vi "Back Right Wheel.vi"(9 "output cluster 2":T2, 10 "Pot Val in":dbl, 11 "Wheel Angle Offset":dbl) -> (0 "Wheel Angle":dbl, 1 "Drive Speed":dbl, 3 "Wheel Speed":dbl)   [LabVIEW 2019]
uses:
  <vilib>/addons/control/pid/pid.llb/PID (DBL).vi
  <vilib>/addons/control/pid/NI_PID_pid.lvlib
panel:
  in  "PID gains":T1={"proportional gain (Kc)"=0.01, "integral time (Ti, min)"=0.0, "derivative time (Td, min)"=0.0} {"derivative time (Td, min)" format="%.3f"; "integral time (Ti, min)" format="%.3f"; "proportional gain (Kc)" format="%.3f"}
  out "Requested Angle":dbl
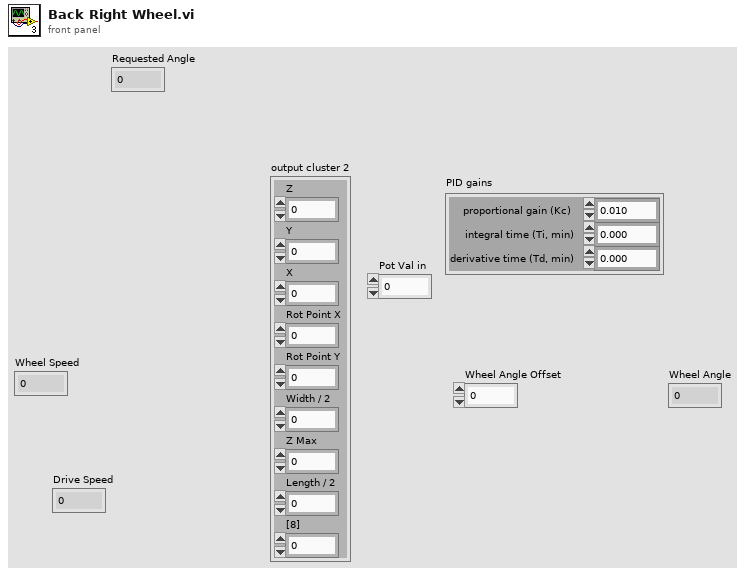
[diagram p1: front panel]
types:
  T1 = cluster{"proportional gain (Kc)":dbl, "integral time (Ti, min)":dbl, "derivative time (Td, min)":dbl}
  T2 = cluster{"Z":dbl, "Y":dbl, "X":dbl, "Rot Point X":dbl, "Rot Point Y":dbl, "Width / 2":dbl, "Z Max":dbl, "Length / 2":dbl, "[8]":dbl}
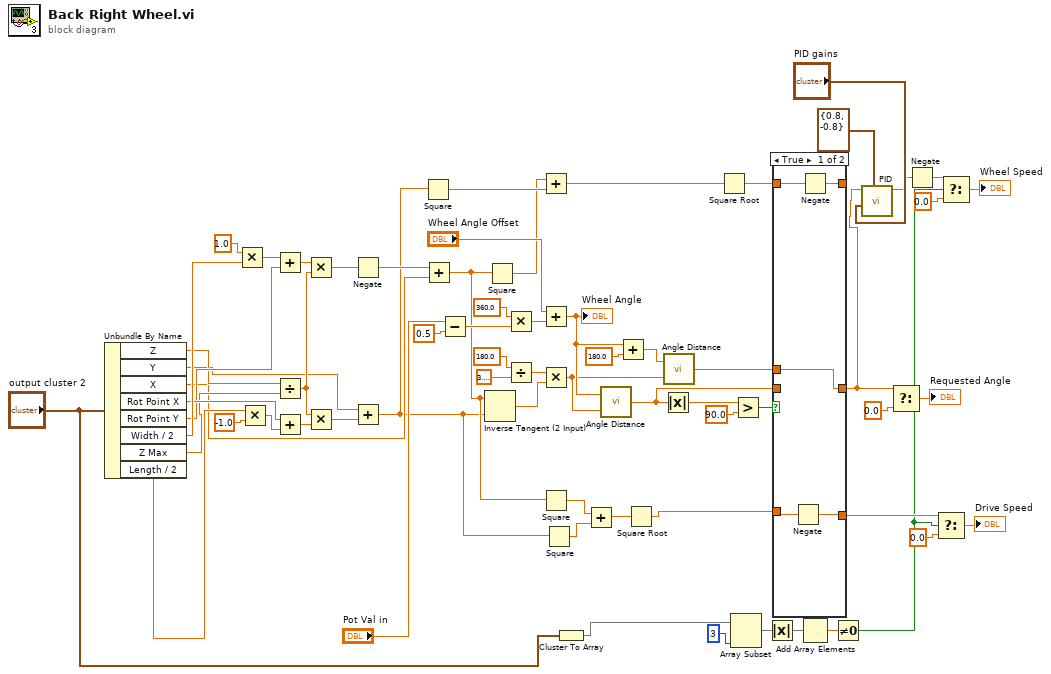
[diagram p0: block diagram]
diagram:
  n1 = Unbundle By Name("output cluster 2") -> ("Z"=w21:dbl, "Y"=w19:dbl, "X"=w18:dbl, "Rot Point X"=w23:dbl, "Rot Point Y"=w22:dbl, "Width / 2"=w63:dbl, "Z Max"=w20:dbl, "Length / 2"=w64:dbl)
  n2 = Multiply(x=1.0, y=w63) -> (x*y=w34:dbl)
  n3 = Multiply(x=w64, y=-1.0) -> (x*y=w33:dbl)
  n4 = Add(x=w34, y=w22) -> (x+y=w35:dbl)
  n5 = Divide(x=w21, y=w20) -> (x/y=w40:dbl)
  n6 = Add(x=w23, y=w33) -> (x+y=w41:dbl)
  n7 = Multiply(x=w35, y=w40) -> (x*y=w37:dbl)
  n8 = Multiply(x=w40, y=w41) -> (x*y=w38:dbl)
  n9 = Negate(x=w37) -> (-x=w36:dbl)
  n10 = Add(x=w19, y=w38) -> (x+y=w5:dbl)
  n11 = Square(x=w5) -> (x^2=w50:dbl)
  n12 = Add(x=w36, y=w18) -> (x+y=w6:dbl)
  n13 = Subtract(x="Pot Val in", y=0.5) -> (x-y=w61:dbl)
  n14 = Inverse Tangent (2 Input)(1:w5, 2:w6) -> (0:w51:dbl)
  n15 = Square(x=w6) -> (x^2=w39:dbl)
  n16 = Multiply(x=360.0 ("y"), y=w61) -> (x*y=w59:dbl)
  n17 = Divide(x=180.0 ("y"), y=3.141592653589793) -> (x/y=w48:dbl)
  n18 = Add(x=w39, y=w50) -> (x+y=w49:dbl)
  n19 = Add(x="Wheel Angle Offset", y=w59) -> (x+y=w54:dbl)
  "Wheel Angle" <- w54
  n20 = Multiply(x=w48, y=w51) -> (x*y=w32:dbl)
  n21 = Square(x=w6) -> (x^2=w12:dbl)
  n22 = Square(x=w5) -> (x^2=w11:dbl)
  n23 = Cluster To Array(cluster="output cluster 2") -> (array=w17:dbl[])
  n24 = Add(x=w12, y=w11) -> (x+y=w13:dbl)
  n25 = call "Angle Distance.vi"("target angle"=w32, "current angle"=w54) -> ("distance"=w27:dbl)
  n26 = Add(x=w54, y=180.0) -> (x+y=w55:dbl)
  n27 = Square Root(x=w13) -> (sqrt(x)=w7:dbl)
  n28 = Absolute Value(x=w27) -> (abs(x)=w30:dbl)
  n29 = call "Angle Distance.vi"("target angle"=w32, "current angle"=w55) -> ("distance"=w28:dbl)
  n30 = Square Root(x=w49) -> (sqrt(x)=w26:dbl)
  n31 = Array Subset(array=w17, length=3) -> (w45:dbl[])  [unwired: 1 in]
  n32 = Greater?(x=w30, y=90.0) -> (0:w29:bool)
  n33 = Absolute Value(x=w45) -> (abs(x)=w42:dbl[])
  n34 = case shown="True" w29 {
    tunnel: w28 -> [w69 _]
    tunnel: w27 -> [_ w74]
    tunnel: [w70 w73] -> _
    tunnel: w26 -> [w71 w73]
    tunnel: [w69 w74] -> w3
    tunnel: [w68 w72] -> w8
    tunnel: w7 -> [w67 w72]
    frame True {
      n35 = Negate(x=w67) -> (-x=w68:dbl)
      n36 = Negate(x=w71) -> (-x=w70:dbl)
    }
    frame False {
    }
  }
  n37 = Add Array Elements(numeric array=w42) -> (sum=w52:dbl)
  n38 = Not Equal To 0?(x=w52) -> (x != 0?=w4:bool)
  n39 = call-poly <vilib>:"PID.vi"("output range"=cluster{"output high":dbl, "output low":dbl} {"output high"=0.8, "output low"=-0.8}, "PID gains"="PID gains", "setpoint"=w3) -> ("output"=w1:dbl)  [unwired: 7 in, 1 out]
  n40 = Select(t=w3, s=w4, f=0.0) -> (s? t:f=→"Requested Angle":dbl)
  n41 = Negate(x=w1) -> (-x=w2:dbl)
  n42 = Select(t=w8, s=w4, f=0.0) -> (s? t:f=→"Drive Speed":dbl)
  n43 = Select(t=w2, s=w4, f=0.0) -> (s? t:f=→"Wheel Speed":dbl)
